vi "TDMS GET DATA.vi"(5 "offset":i32, 7 "Grupo":string, 8 "error in":errorcluster, 10 "channel name(s) in":string, 11 "file path":path) -> (0 "error out":errorcluster, 2 "lengh":i32, 3 "transposed array":string[][](array[string]))   [LabVIEW 2015]
panel:
  out "data 2":timestamp[](array[timestamp])
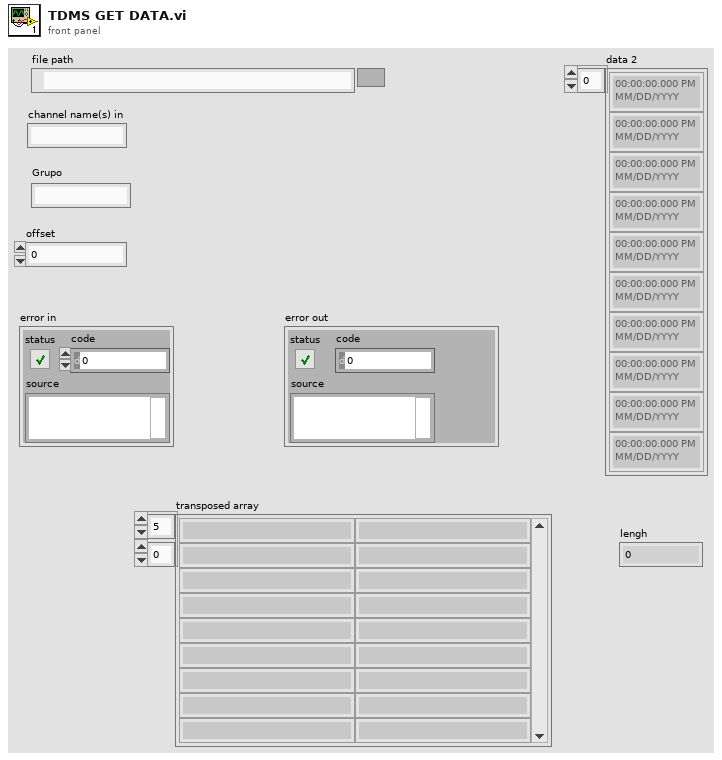
[diagram p1: front panel]
types:
  T1 = enum16{"open", "open or create", "create or replace", "create", "open (read-only)"}
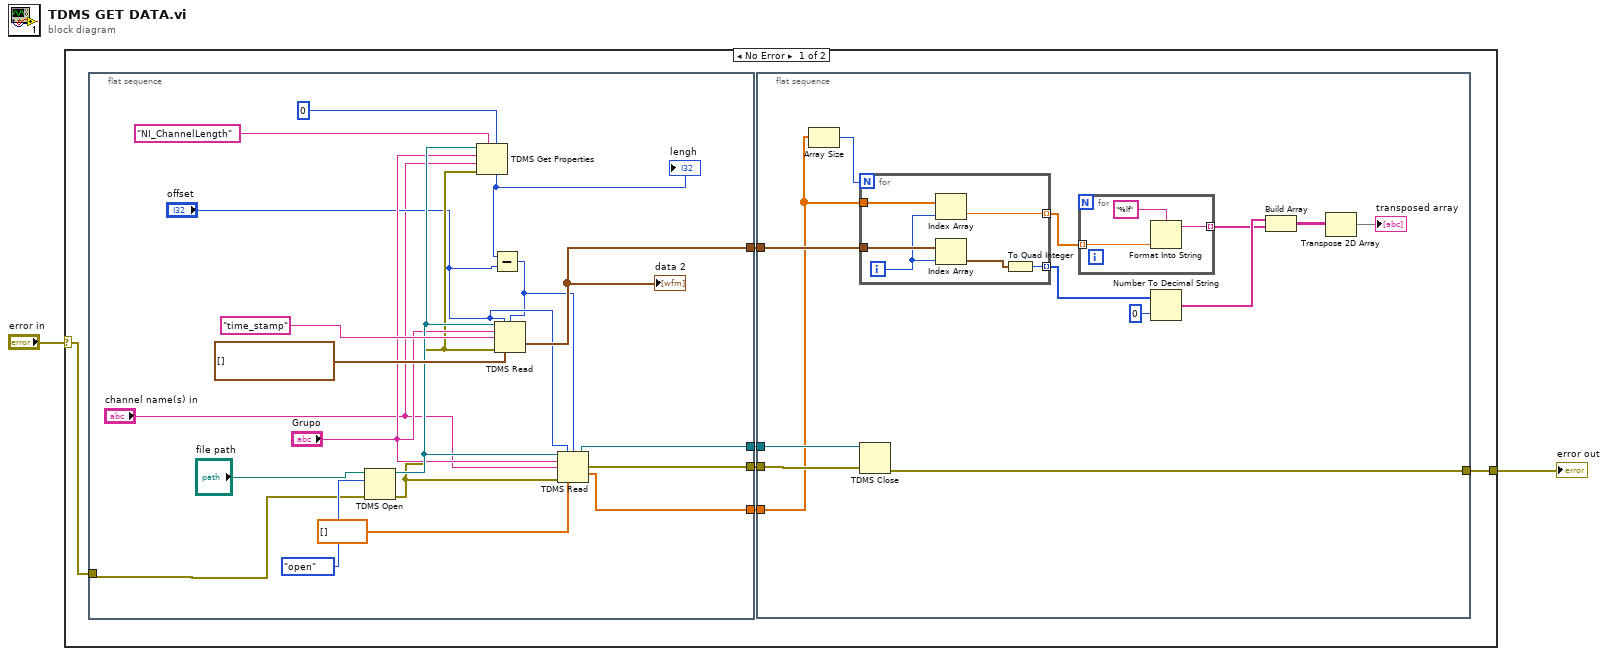
[diagram p0: block diagram]
diagram:
  n1 = case shown="No Error" "error in" {
    selector: "error in" -> [w3 w50]
    tunnel: [w4 w50] -> w1
    frame No Error {
      n2 = flat-sequence {
        tunnel: [w48] -> w8
        tunnel: [w47] -> w7
        tunnel: [w33] -> w6
        tunnel: [w38] -> w5
        tunnel: w3 -> [w31]
        frame #0 {
          n3 = TDMS Open(8:w31, 10:T1."open" ("operation (0:open)"), 11:"file path") -> (0:w39:errorcluster, 3:w41:refnum<k34>)  [unwired: 4 in]
          n4 = TDMS Get Properties(5:0, 7:"NI_ChannelLength" ("property name"), 8:w39, 9:"channel name(s) in", 10:"Grupo", 11:w41) -> (4:w37:i32)  [unwired: 5 out]
          "lengh" <- w37
          n5 = Subtract(x=w37, y="offset") -> (x-y=w35:i32)
          n6 = TDMS Read(0:w41, 1:"offset", 2:w35, 5:"Grupo", 7:"time_stamp", 11:w39, 12:timestamp[] []) -> (10:w38:timestamp[])  [unwired: 1 in, 5 out]
          "data 2" <- w38
          n7 = TDMS Read(0:w41, 1:"offset", 2:w35, 5:"Grupo", 7:"channel name(s) in", 11:w39, 12:dbl[] []) -> (4:w48:refnum<k34>, 10:w33:dbl[], 15:w47:errorcluster)  [unwired: 1 in, 3 out]
        }
      }
      n8 = flat-sequence {
        tunnel: w8 -> [w21]
        tunnel: w7 -> [w20]
        tunnel: w6 -> [w16]
        tunnel: w5 -> [w19]
        tunnel: [w11] -> w4
        frame #0 {
          n9 = Array Size(array=w16) -> (size(s)=w15:i32)
          n10 = for {
            N: w15 -> [_]
            tunnel: w16 -> [w30]
            tunnel: w19 -> [w29]
            tunnel: [w27] -> w13 mode=indexing
            tunnel: [w25] -> w9 mode=indexing
            i -> [w28]
            n11 = Index Array(array=w30, index=w28) -> (element=w27:dbl)
            n12 = Index Array(array=w29, index=w28) -> (element=w26:timestamp)
            n13 = To Quad Integer(1:w26) -> (0:w25:i64)
          }
          n14 = TDMS Close(8:w20, 11:w21) -> (0:w11:errorcluster)  [unwired: 1 out]
          n15 = for {
            tunnel: w13 -> [w24] mode=indexing
            tunnel: [w23] -> w12 mode=indexing
            n16 = Format Into String(format string="%lf", w24) -> (resulting string=w23:string)  [unwired: 2 in, 1 out]
          }
          n17 = Number To Decimal String(number=w9, width (-)=i16 0) -> (decimal integer string=w17:string[])
          n18 = Build Array(w17, w12) -> (w18:string[][])
          n19 = Transpose 2D Array(2D array=w18) -> (transposed array=→"transposed array":string[][])
        }
      }
    }
    frame Error {
    }
  }
  "error out" <- w1
